vi "Read Data.vi"   [LabVIEW 2019, in "D2XX-lv.lvlib"]
doc: "Read data from an open device."
uses:
  D2XX-lv.lvlib
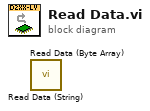
[diagram p0: block diagram]
diagram:
  n1 = call "Read Data (String).vi"() -> ()  [unwired: 8 in, 4 out]
  n2 = call "Read Data (Byte Array).vi"() -> ()  [unwired: 8 in, 4 out]
